vi "Test 1 Correct Command is Sent on Read Voltage.vi"(8 "error in (no error)":errorcluster, 11 "Test Case In":refnum<class "Driver Test.lvclass">) -> (0 "error out":errorcluster, 3 "Test Case Out":refnum<class "Driver Test.lvclass">)   [LabVIEW 2020, in "Driver Test.lvclass"]
uses:
  Driver Test.lvclass
  C:/Program Files (x86)/National Instruments/LabVIEW 2020/vi.lib/Astemes/LUnit/Test Case.lvclass
  Mock Serial.lvclass
  C:/Program Files (x86)/National Instruments/LabVIEW 2020/vi.lib/Astemes/LMock/Mock.lvclass
  C:/git/astemes-lmock/sandbox/Examples/Serial/Serial.lvclass/Serial.lvclass
  Driver Test.lvclass/Driver Test.ctl
  Driver/Driver.lvclass
  C:/git/astemes-lmock/sandbox/Examples/Mock Serial.lvclass
  <vilib>/Astemes/LMock/LMock Verifier.lvclass
  <vilib>/Astemes/LMock/One.lvclass
  <vilib>/Astemes/LMock/One/One Identical Inputs.vi
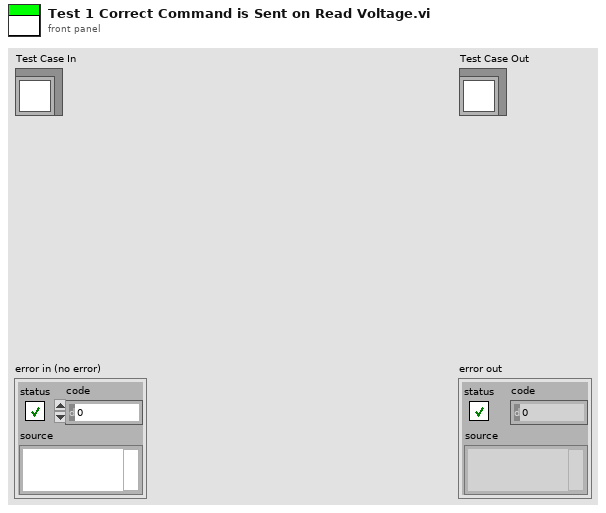
[diagram p1: front panel]
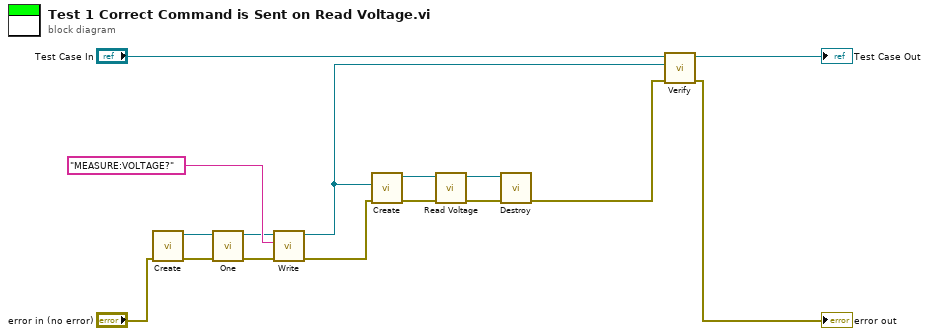
[diagram p0: block diagram]
diagram:
  n1 = call "Create.vi"("error in (no error)"="error in (no error)") -> ("error out"=w6:errorcluster, "Mock Class Generator out"=w2:refnum<class "Mock Serial.lvclass">)  [unwired: 9 in]
  n2 = call-poly <vilib>:"One.vi"("error in (no error)"=w6, "Mock in"=w2) -> ("error out"=w3:errorcluster, "Mock out"=w1:refnum<class "Mock Serial.lvclass">)  [unwired: 8 in]
  n3 = call-dynamic "Write.vi"("error in (no error)"=w3, "write buffer"="MEASURE:VOLTAGE?", "Serial in"=w1) -> ("error out"=w7:errorcluster, "Serial out"=w8:refnum<class "Mock Serial.lvclass">)  [unwired: 6 in, 1 out]
  n4 = call "Create.vi"("error in (no error)"=w7, "Serial"=w8) -> ("error out"=w13:errorcluster, "Driver"=w11:refnum<class "Driver.lvclass">)  [unwired: 8 in]
  n5 = call "Read Voltage.vi"("error in (no error)"=w13, "Driver In"=w11) -> ("error out"=w12:errorcluster, "Driver Out"=w10:refnum<class "Driver.lvclass">)  [unwired: 7 in, 1 out]
  n6 = call "Destroy.vi"("error in (no error)"=w12, "Driver"=w10) -> ("error out"=w5:errorcluster)  [unwired: 9 in]
  n7 = call <vilib>:"Verify.vi"("error in (no error)"=w5, "Mock"=w8, "LUnit Test Case In"="Test Case In") -> ("error out"=→"error out":errorcluster, "LUnit Test Case Out"=→"Test Case Out":refnum<class "Driver Test.lvclass">)  [unwired: 7 in]
